vi "Analyze.vi"(8 "error in (no error)":errorcluster, 10 "Image in":T1, 11 "Analyze Fluence in":refnum<class "Analyze Fluence.lvclass">) -> (0 "error out":errorcluster, 1 "Result":refnum<class "Analyze Results Base.lvclass">, 2 "Image out":T1, 3 "Analyze Fluence out":refnum<class "Analyze Fluence.lvclass">)   [LabVIEW 2020, in "Analyze.lvlib" / "Analyze Fluence.lvclass"]
doc: "In Variant Attributes to provide:\nEnergy: Energy in J\nROI: Image Display ROI Deskriptor\n\nOut Variant Attributes:\nFluence Infos: Array of Fluence Info.ctl\nMax Fluence: Maximal detected Fluence in J/cm^2"
uses:
  Analyze Fluence.lvclass
  C:/POLARIS Programme/POLARIS-AS-3-Cams/Submodules/HIJ Vision/Analyze/Analyze Classes/Analyze BaseClass/Analyze BaseClass/Analyze BaseClass.lvclass
  <vilib>/vision/Image Controls.llb/IMAQ Image.ctl
  Results and Overlays/Results Base/Analyze Results Base.lvclass
  Results and Overlays/Results Fluence/Analyze Results Fluence.lvclass
  C:/POLARIS Programme/POLARIS-AS-3-Cams/Submodules/HIJ Vision/Analyze/Results and Overlays/Results Base/Analyze Results Base.lvclass
  Analyze BaseClass/Analyze BaseClass/Analyze BaseClass.lvclass
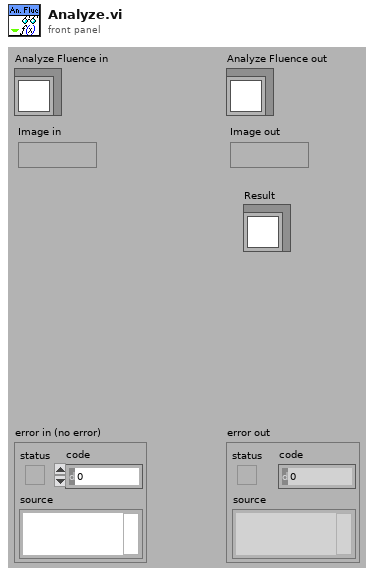
[diagram p1: front panel]
types:
  T1 = typedef "IMAQ Image.ctl" = refnum<image>
  T2 = typedef "Analyze.lvlib/Analyze Fluence.lvclass/Fluence Info.ctl" = cluster{"Fluence J/cm^2":dbl[unit], "Energy in Area":dbl[unit], "max value":i64, "Max fluence area":cluster{"Left":i32, "Top":i32, "Right":i32, "Bottom":i32}}
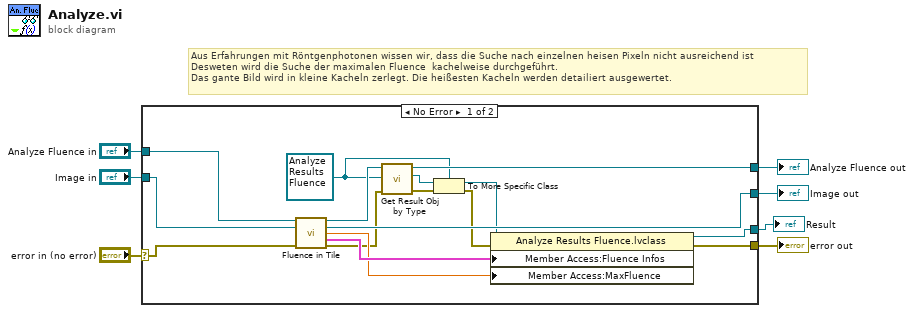
[diagram p0: block diagram]
diagram:
  # "Aus Erfahrungen mit Röntgenphotonen wissen wir, dass die Suche nach einzelnen heisen Pixeln nicht ausreichend ist\nDesweten wird die Suche der maximalen Fluence  kachelweise durchgeführt.\nDas gante Bild wird in kleine Kacheln zerlegt. Die heißesten Kacheln werden detailiert ausgewertet."
  n1 = case shown="No Error" "error in (no error)" {
    selector: "error in (no error)" -> [w16 w25]
    tunnel: [w14 w24] -> w7
    tunnel: [w18 w25] -> w6
    tunnel: "Analyze Fluence in" -> [w22 w24]
    tunnel: "Image in" -> [w17 w26]
    tunnel: [w21 w26] -> w3
    tunnel: [w15 _] -> w1
    frame No Error {
      w13 = refnum<class "Analyze Results Fluence.lvclass"> refnum ("Analyze Results Fluence.lvclass")
      n2 = call "Fluence in Tile.vi"("Analyze Fluence in"=w22, "Image in"=w17, "error in (no error)"=w16) -> ("Analyze Fluence out"=w23:refnum<class "Analyze Fluence.lvclass">, "Image Dst Out"=w21:T1, "Max Fluence"=w19:dbl[unit], "fluence infos"=w20:T2[], "error out"=w8:errorcluster)  [unwired: 8 in]
      n3 = call "Get Result Obj by Type.vi"("error in (no error)"=w8, "Parameter Type"=w13, "Analyze BaseClass in"=w23) -> ("error out"=w9:errorcluster, "Parameter"=w12:refnum<class "Analyze Results Base.lvclass">, "Analyze BaseClass out"=w14:refnum<class "Analyze Fluence.lvclass">)  [unwired: 5 in, 1 out]
      n4 = To More Specific Class(target class=w13, reference=w12, error in=w9) -> (specific class reference=w11:refnum<class "Analyze Results Fluence.lvclass">, error out=w10:errorcluster)
      n5 = property class="Analyze Results Fluence.lvclass"(reference=w11, error in=w10, "Member Access:Fluence Infos"=w20, "Member Access:MaxFluence"=w19) -> (reference out=w15:refnum<class "Analyze Results Fluence.lvclass">, error out=w18:errorcluster)
    }
    frame Error {
    }
  }
  "error out" <- w6
  "Analyze Fluence out" <- w7
  "Image out" <- w3
  "Result" <- w1
